vi "JSON.vi"(8 "error in (no error)":errorcluster, 11 "RJSONDebug in":refnum<class "RJSONDebug.lvclass">) -> (0 "error out":errorcluster, 2 "JSON":string, 3 "RJSONDebug out":refnum<class "RJSONDebug.lvclass">)   [LabVIEW 2020, in "obs-websocket.lvlib" / "RJSONDebug.lvclass"]
uses:
  RJSONDebug.lvclass
  RJSONDebug.lvclass/RJSONDebug.ctl
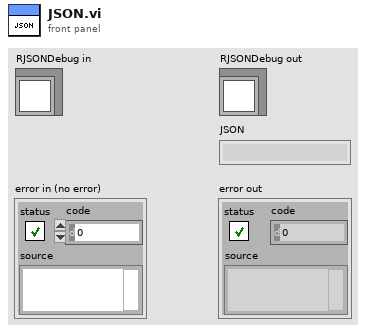
[diagram p1: front panel]
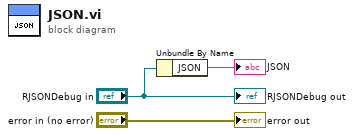
[diagram p0: block diagram]
diagram:
  n1 = Unbundle By Name("RJSONDebug in") -> ("JSON"=→"JSON":string)
  "error out" <- "error in (no error)"
  "RJSONDebug out" <- "RJSONDebug in"
